vi "ESP32 Continuous Serial Write and Read.vi"() -> ()   [LabVIEW 2025]
doc: "This example performs writes and reads on a serial port, as directed by the user. You can press the Write and Read buttons, and change the Read Count, while the example is running.\n\nThe parameters set for the serial port must match the parameters of the connected instrument or device. In this example, the Read Count parameter specifies the number of bytes that the serial port reads. If there were more bytes at the port than the specified number, those bytes would not be read. If there were less bytes at the port than the specified number, you would receive a timeout error.\n\nThis example expands upon the flow control options for XON and XOFF, allowing the user to choose those control characters. Also, the user can enable or disable a termination character. Some devices require a termination character in order to identify the end of command strings. Some devices send a termination character to signify the end of data to be read. This example shows how you can end the Read operation once a termination character is detected in the buffer and/or append a termination character at the end of the Write data."
uses:
  Serial - Settings.ctl
  Control 1.ctl
  ESP32-PSOC-State Machine-1.ctl
  <vilib>/Instr/_visa.llb/VISA Flush IO Buffer Mask.ctl
  <vilib>/Instr/_visa.llb/VISA Configure Serial Port (Instr).vi
panel:
  in  "Command R":bool
  out "error":bool
  out "Connected":bool
  out "Serial Settings:Number of Bytes at Serial Port":u32
  out "Response 2":string
  in  "Command B":bool
  in  "Command A":bool
  in  "Toggle LED":bool
  in  "Enum":T1
  in  "Termination Character":u8=10 format="%.0x"
  in  "End Write on Termination Character?":bool=TRUE
  in  "Stop":bool
  out "Read Count":u32=1000
  out "Response":string
  in  "XON/XOFF Characters":T2={"XON"=enum."DC1", "XOFF"=enum."DC3"}
  in  "Serial Settings":T3={"baud rate"=115200, "data bits"=8, "parity"=enum."None", "stop bits"=10, "flow control"=0} {"flow control" items=["None"=0, "XON/XOFF"=1, "RTS/CTS"=2, "DTR/DSR"=4]; "stop bits" items=["1.0"=10, "1.5"=15, "2.0"=20]; "data bits" min=5 max=8 step=1; "baud rate" items=["75"=75, "110"=110, "134"=134, "150"=150, "300"=300, "600"=600, "1200"=1200, "1800"=1800, "2400"=2400, "4800"=4800, "7200"=7200, "9600"=9600, "14400"=14400, "19200"=19200, "28800"=28800, "38400"=38400, "56000"=56000, "57600"=57600, "115200"=115200, "128000"=128000, "230400"=230400]}
  in  "End Read on Termination Character?":bool=TRUE
  in  "VISA resource name":refnum<visa-resource-name>="COM3"
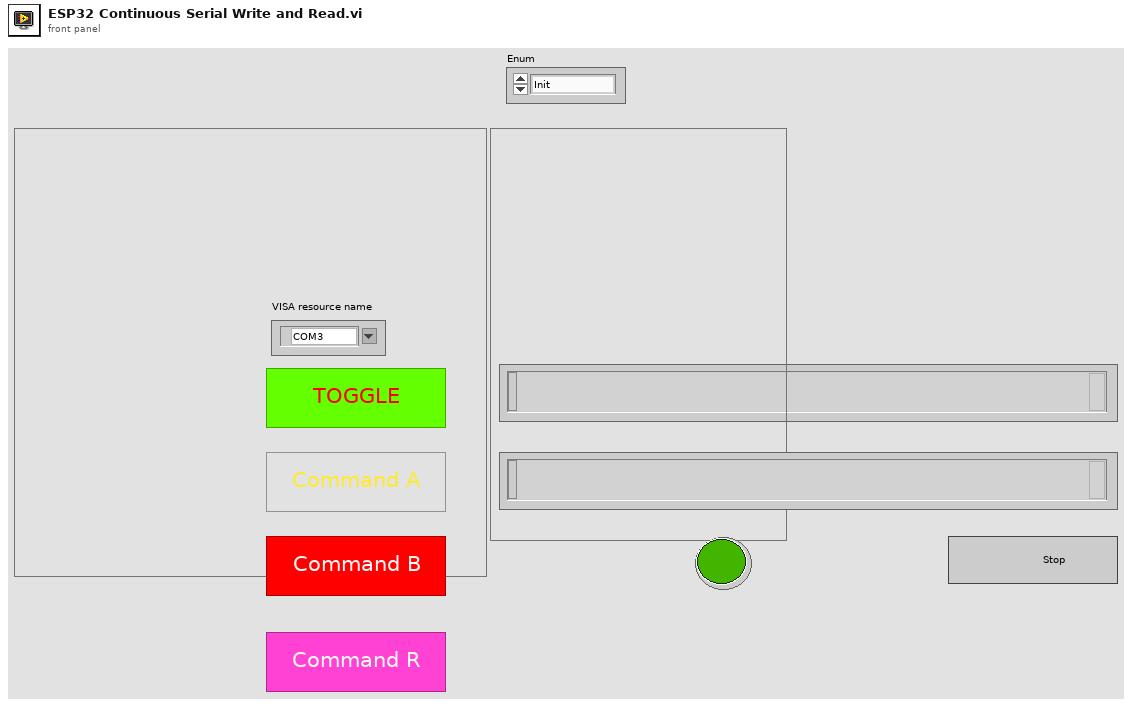
[diagram p1: front panel]
types:
  T1 = typedef "ESP32-PSOC-State Machine-1.ctl" = enum8{"Init", "Connect", "idle", "send", "wait", "receive", "que", "error", "exit"}
  T2 = typedef "Control 1.ctl" = cluster{"XON":enum16{"NUL", "SOH", "STX", "ETX", "EOT", "ENQ", "ACK", "BEL", "BS", "HT", "LF", "VT", "FF", "CR", "SO", "SI", "DLE", "DC1", "DC2", "DC3", "DC4", "NAK", "SYN", "ETB", "CAN", "EM", "SUB", "ESC", "FS", "GS", "RS", "US", "SP", "!", "\"", "#", "$", "%", "&", "'", "(", ")", "*", "+", ",", "- (-)", ".", "/", "0", "1", "2", "3", "4", "5", "6", "7", "8", "9", ":", ";", "<", "=", ">", "?", "@", "A", "B", "C", "D", "E", "F", "G", "H", "I", "J", "K", "L", "M", "N", "O", "P", "Q", "R", "S", "T", "U", "V", "W", "X", "Y", "Z", "[", "\\", "]", "^", "_", "`", "a", "b", "c", "d", "e", "f", "g", "h", "i", "j", "k", "l", "m", "n", "o", "p", "q", "r", "s", "t", "u", "v", "w", "x", "y", "z", "{", "|", "}", "~"}, "XOFF":enum16{"NUL", "SOH", "STX", "ETX", "EOT", "ENQ", "ACK", "BEL", "BS", "HT", "LF", "VT", "FF", "CR", "SO", "SI", "DLE", "DC1", "DC2", "DC3", "DC4", "NAK", "SYN", "ETB", "CAN", "EM", "SUB", "ESC", "FS", "GS", "RS", "US", "SP", "!", "\"", "#", "$", "%", "&", "'", "(", ")", "*", "+", ",", "- (-)", ".", "/", "0", "1", "2", "3", "4", "5", "6", "7", "8", "9", ":", ";", "<", "=", ">", "?", "@", "A", "B", "C", "D", "E", "F", "G", "H", "I", "J", "K", "L", "M", "N", "O", "P", "Q", "R", "S", "T", "U", "V", "W", "X", "Y", "Z", "[", "\\", "]", "^", "_", "`", "a", "b", "c", "d", "e", "f", "g", "h", "i", "j", "k", "l", "m", "n", "o", "p", "q", "r", "s", "t", "u", "v", "w", "x", "y", "z", "{", "|", "}", "~"}}
  T3 = typedef "Serial - Settings.ctl" = cluster{"baud rate":u32, "data bits":u16, "parity":enum16{"None", "Odd", "Even", "Mark", "Space"}, "stop bits":u16, "flow control":u16}
  T4 = enum16{"NUL", "SOH", "STX", "ETX", "EOT", "ENQ", "ACK", "BEL", "BS", "HT", "LF", "VT", "FF", "CR", "SO", "SI", "DLE", "DC1", "DC2", "DC3", "DC4", "NAK", "SYN", "ETB", "CAN", "EM", "SUB", "ESC", "FS", "GS", "RS", "US", "SP", "!", "\"", "#", "$", "%", "&", "'", "(", ")", "*", "+", ",", "- (-)", ".", "/", "0", "1", "2", "3", "4", "5", "6", "7", "8", "9", ":", ";", "<", "=", ">", "?", "@", "A", "B", "C", "D", "E", "F", "G", "H", "I", "J", "K", "L", "M", "N", "O", "P", "Q", "R", "S", "T", "U", "V", "W", "X", "Y", "Z", "[", "\\", "]", "^", "_", "`", "a", "b", "c", "d", "e", "f", "g", "h", "i", "j", "k", "l", "m", "n", "o", "p", "q", "r", "s", "t", "u", "v", "w", "x", "y", "z", "{", "|", "}", "~"}
  T5 = typedef "VISA Flush IO Buffer Mask.ctl" = u16
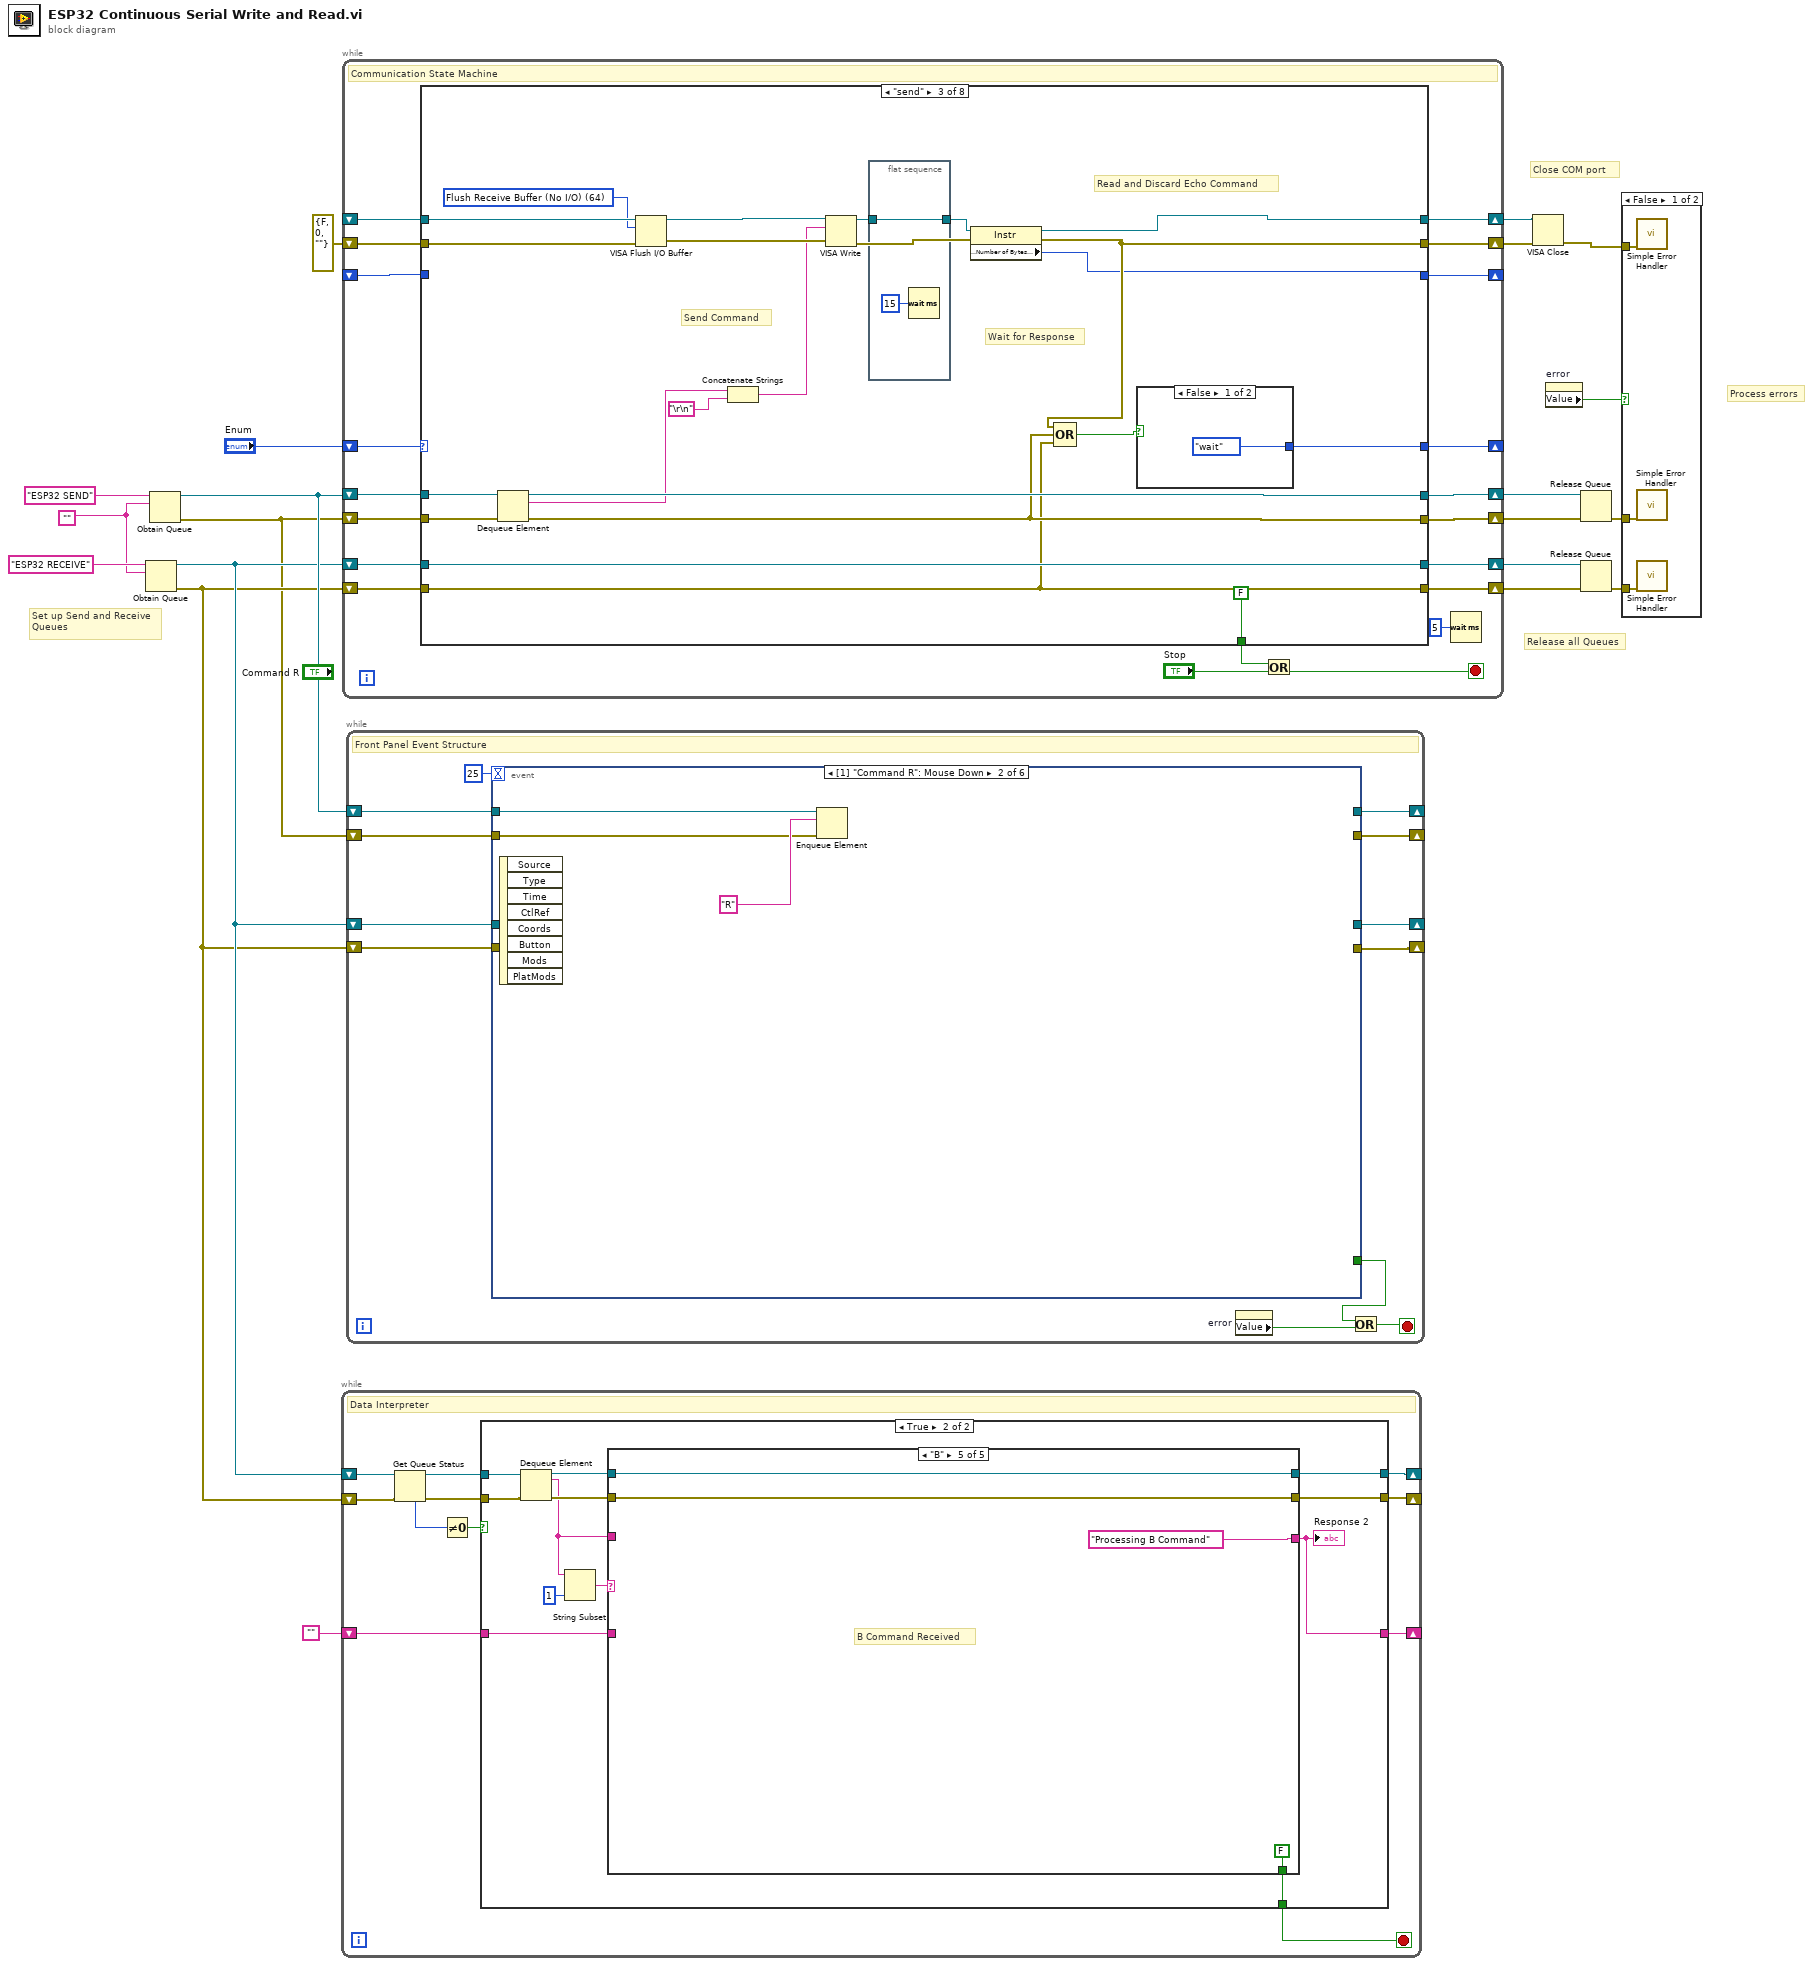
[diagram p0: block diagram]
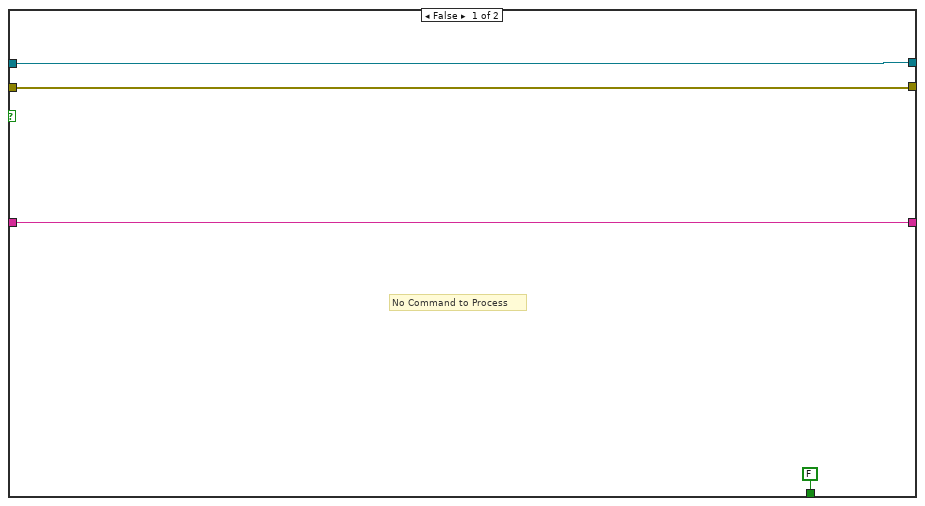
[diagram p3: hidden frame]
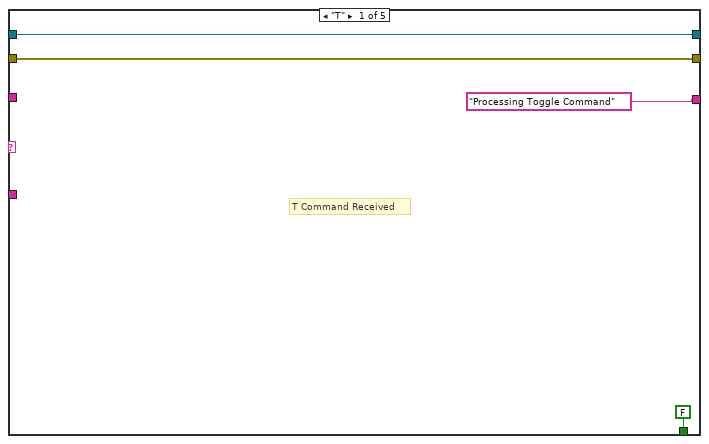
[diagram p4: hidden frame]
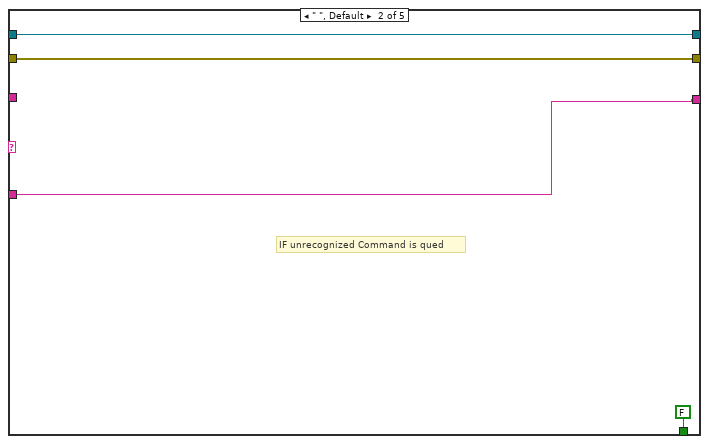
[diagram p5: hidden frame]
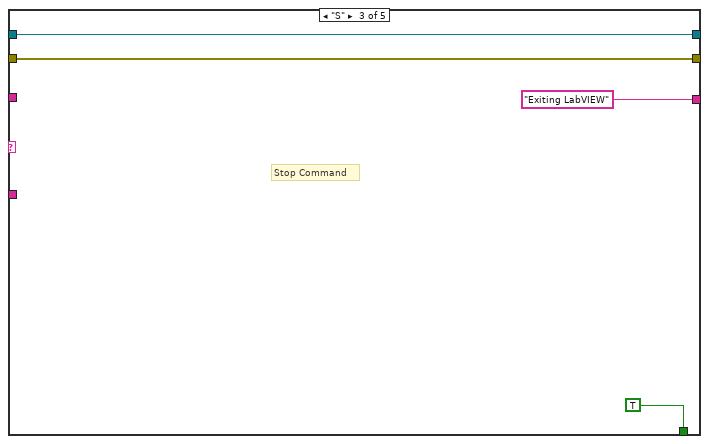
[diagram p6: hidden frame]
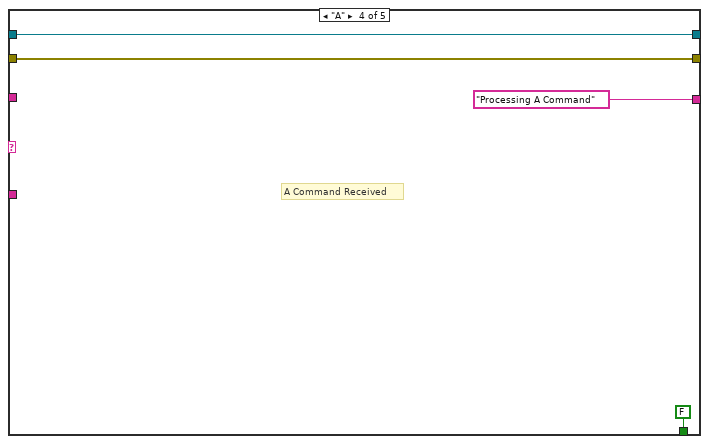
[diagram p7: hidden frame]
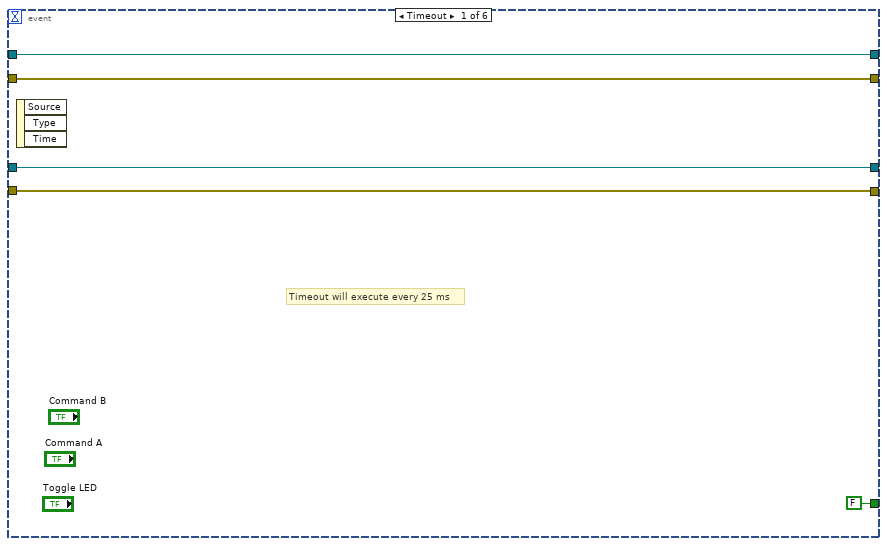
[diagram p8: hidden frame]
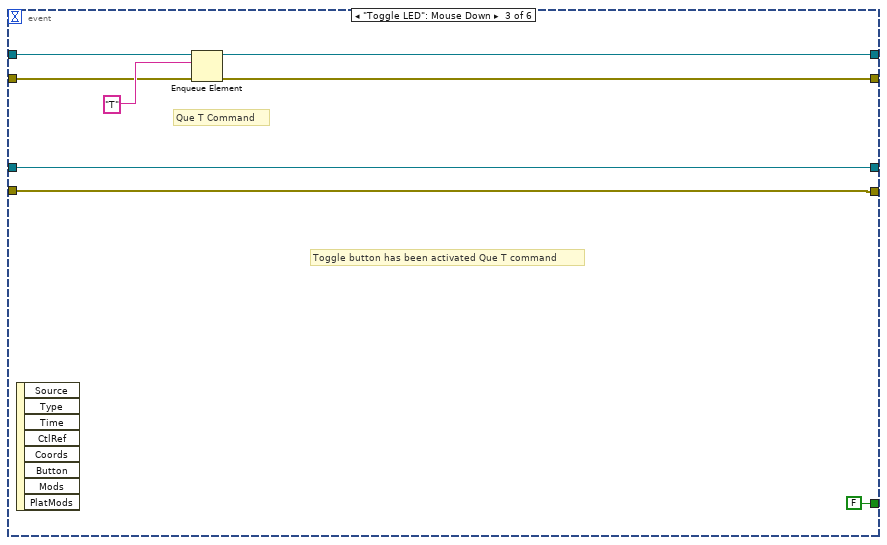
[diagram p9: hidden frame]
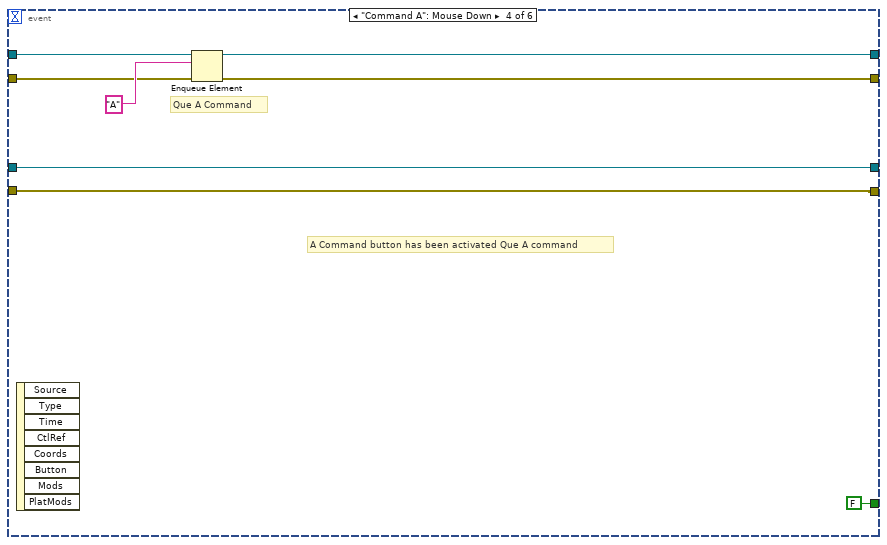
[diagram p10: hidden frame]
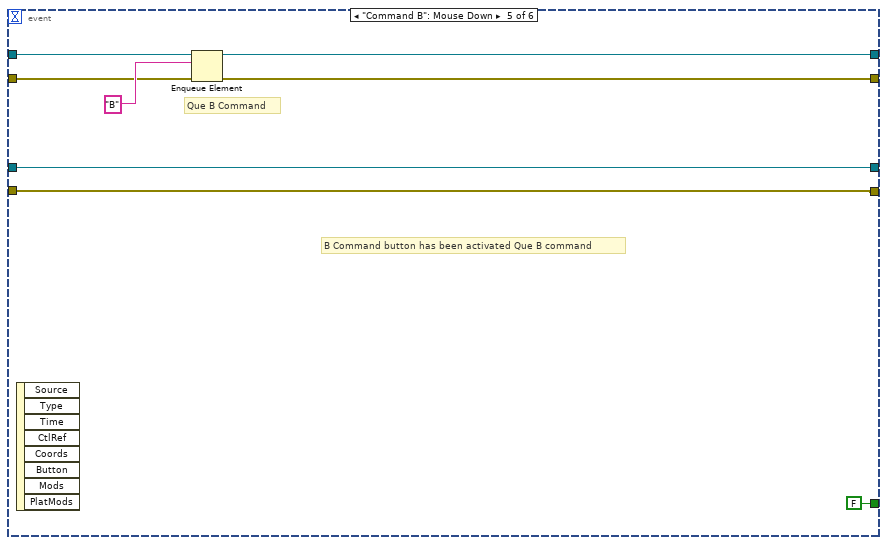
[diagram p11: hidden frame]
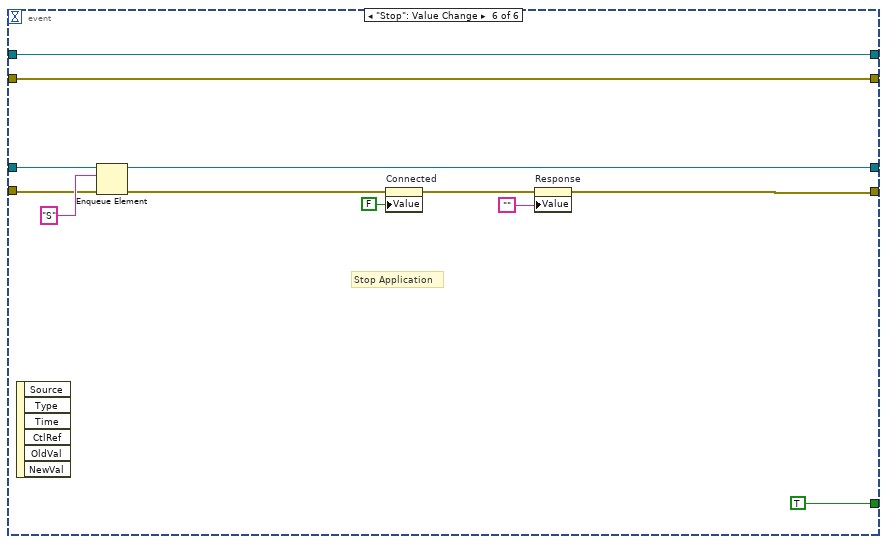
[diagram p12: hidden frame]
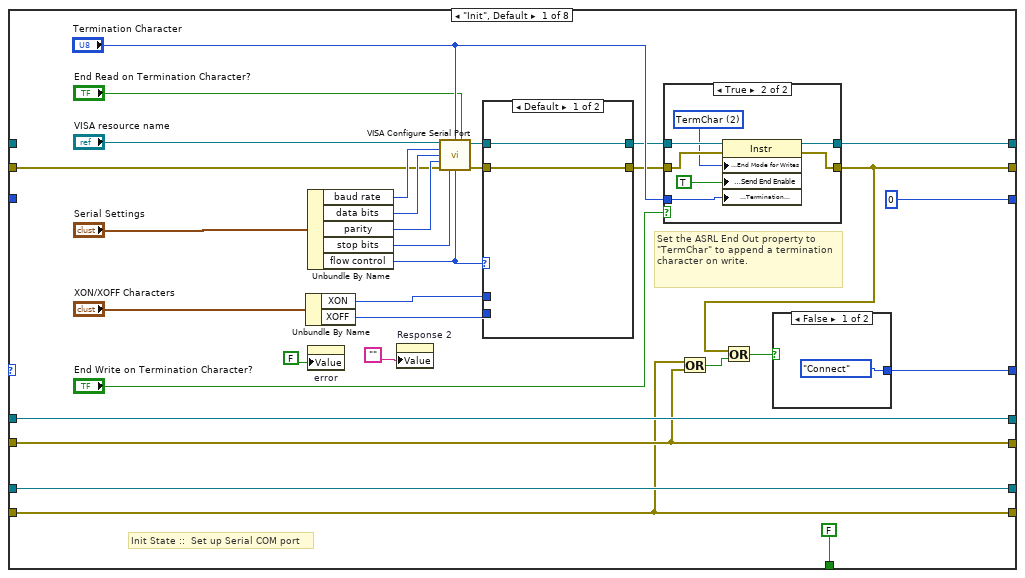
[diagram p13: hidden frame]
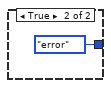
[diagram p14: hidden frame]
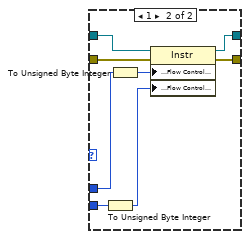
[diagram p16: hidden frame]
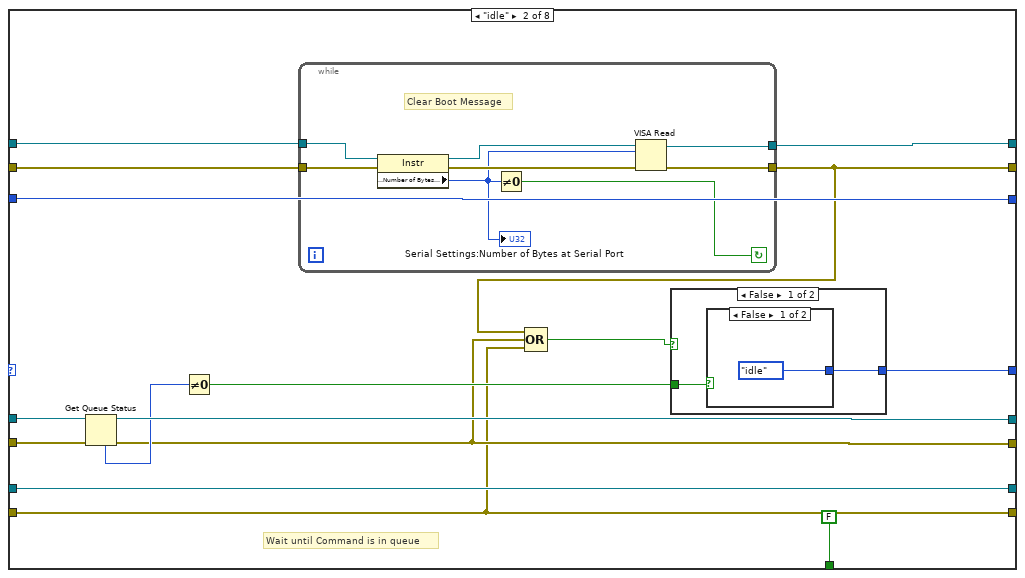
[diagram p17: hidden frame]
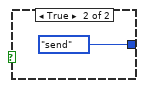
[diagram p18: hidden frame]
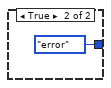
[diagram p19: hidden frame]
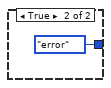
[diagram p20: hidden frame]
diagram:
  w10 = ""
  # "Process errors"
  # "Release all Queues"
  # "Close COM port"
  # "Set up Send and Receive\nQueues"
  n1 = Obtain Queue(name (unnamed)="ESP32 RECEIVE", element data type=w10) -> (queue out=w9:refnum<queue>, error out=w8:errorcluster)  [unwired: 3 in, 1 out]
  n2 = Obtain Queue(name (unnamed)="ESP32 SEND", element data type=w10) -> (queue out=w12:refnum<queue>, error out=w2:errorcluster)  [unwired: 3 in, 1 out]
  n3 = while {
    shift-right: [w25] -> _
    shift-left: w9 -> [w31]
    shift-right: [w24] -> _
    shift-left: w8 -> [w30]
    shift-right: [w22] -> _
    shift-left: "" -> [w21]
    stop <- w23 stop-if-true
    # "Data Interpreter"
    n4 = Get Queue Status(queue=w31, error in (no error)=w30) -> (queue out=w27:refnum<queue>, error out=w26:errorcluster, # elements in queue=w29:i32)  [unwired: 1 in, 5 out]
    n5 = Not Equal To 0?(x=w29) -> (x != 0?=w28:bool)
    n6 = case shown="True" w28 {
      tunnel: w27 -> [w35 w47]
      tunnel: w26 -> [w34 w46]
      tunnel: [w35 w41] -> w25
      tunnel: [w34 w40] -> w24
      tunnel: [FALSE w39] -> w23
      tunnel: [w32 w37] -> w22
      tunnel: w21 -> [w32 w36]
      frame False {
        # "No Command to Process"
      }
      frame True {
        n7 = Dequeue Element(queue=w47, error in (no error)=w46) -> (queue out=w45:refnum<queue>, element=w38:string, error out=w44:errorcluster)  [unwired: 1 in, 1 out]
        n8 = String Subset(string=w38, length (rest)=1 ("length (rest)")) -> (substring=w42:string)  [unwired: 1 in]
        n9 = case shown="\"B\"" w42 {
          tunnel: w45 -> [w51 w55 w59 w63 w67]
          tunnel: w44 -> [w50 w54 w58 w62 w66]
          tunnel: [w51 w55 w59 w63 w67] -> w41
          tunnel: [w50 w54 w58 w62 w66] -> w40
          tunnel: w38 -> [_ _ _ _ _]
          tunnel: [FALSE FALSE TRUE FALSE FALSE] -> w39
          tunnel: ["Processing Toggle Command" w52 "Exiting LabVIEW" "Processing A Command" "Processing B Command"] -> w37
          tunnel: w36 -> [_ w52 _ _ _]
          frame "T" {
            # "T Command Received"
          }
          frame " ", Default {
            # "IF unrecognized Command is qued"
          }
          frame "S" {
            # "Stop Command"
          }
          frame "A" {
            # "A Command Received"
          }
          frame "B" {
            # "B Command Received"
          }
        }
        "Response 2" <- w37
      }
    }
  }
  n10 = while {
    shift-right: [w79] -> w20
    shift-left: w12 -> [w87]
    shift-right: [w78] -> w18
    shift-left: w2 -> [w86]
    shift-right: [w77] -> w19
    shift-left: w9 -> [w85]
    shift-right: [w76] -> w15
    shift-left: w8 -> [w84]
    shift-right: [w71] -> _
    shift-left: "Enum" -> [w70]
    shift-right: [w83] -> w14
    shift-left: _ -> [w80]
    shift-right: [w82] -> w13
    shift-left: errorcluster {"status"=FALSE, "code"=0, "source"=""} ("error out") -> [w81]
    shift-right: [w75] -> _
    shift-left: _ -> [w74]
    stop <- w69 stop-if-true
    # "Communication State Machine"
    n11 = case shown="\"send\"" w70 {
      selector: w70 -> [_ _ _ _ _ _ w282 _]
      tunnel: [w117 w153 w189 w206 w244 w266 w281 w304] -> w79
      tunnel: [w91 w143 w181 w200 w227 w263 w280 w303] -> w78
      tunnel: [w97 w151 w182 w209 w245 ESP32-PSOC-State_Machine-1."exit" ("Enum") w282 ESP32-PSOC-State_Machine-1."idle" ("Enum")] -> w71
      tunnel: w87 -> [w117 w155 w191 w206 w244 w266 w281 w304]
      tunnel: w86 -> [w91 w154 w190 w200 w227 w263 w280 w303]
      tunnel: w85 -> [w118 w149 w188 w203 w239 w265 w279 w302]
      tunnel: w84 -> [w90 w142 w180 w199 w226 w262 w270 w301]
      tunnel: [w99 w146 w177 w208 w235 w268 w285 w306] -> w83
      tunnel: [w93 w144 w175 w201 w228 w264 w284 w307] -> w82
      tunnel: w81 -> [w95 w145 w185 w207 w230 w264 w284 w308]
      tunnel: w80 -> [_ w147 w187 w197 w242 w268 w285 w309]
      tunnel: [w118 w149 w188 w203 w237 w265 w277 w302] -> w77
      tunnel: [w90 w142 w180 w199 w238 w262 w273 w301] -> w76
      tunnel: [u32 0 ("Bytes at Port") w148 w169 w205 w240 w267 w283 w305] -> w75
      tunnel: w74 -> [_ w148 _ _ w218 w267 w283 w305]
      tunnel: [FALSE FALSE FALSE FALSE FALSE FALSE TRUE FALSE] -> w68
      frame "Init", Default {
        # "Init State ::  Set up Serial COM port"
        # "Set the ASRL End Out property to \"TermChar\" to append a termination character on write."
        n12 = Unbundle By Name("XON/XOFF Characters") -> ("XON"=w111:T4, "XOFF"=w112:T4)
        n13 = Unbundle By Name("Serial Settings") -> ("baud rate"=w107:u32, "data bits"=w106:u16, "parity"=w105:enum16{"None", "Odd", "Even", "Mark", "Space"}, "stop bits"=w104:u16, "flow control"=w110:u16)
        n14 = property on="error" class="Bool (strict)"("Value"=FALSE ("error")) -> ()  [unwired: 2 in, 2 out]
        n15 = property on="Response 2" class="Str"("Value"="") -> ()  [unwired: 2 in, 2 out]
        n16 = call-poly "VISA Configure Serial Port"("VISA resource name"="VISA resource name", "termination char\n(0xA = '\\n' = LF)"="Termination Character", "Enable Termination\nChar (T)"="End Read on Termination Character?", "baud rate (9600)"=w107, "data bits (8)"=w106, "parity (0:none)"=w105, "error in (no error)"=w95, "stop bits (10: 1 bit)"=w104, "flow control (0:none)"=w110) -> ("VISA resource name out"=w103:refnum<visa-resource-name>, "error out"=w102:errorcluster)  [unwired: 1 in, 4 out]
        n17 = case shown="Default" w110 {
          tunnel: [w130 w139] -> w113
          tunnel: [w131 w138] -> w114
          tunnel: w102 -> [w130 w137]
          tunnel: w103 -> [w131 w136]
          tunnel: w111 -> [_ w135]
          tunnel: w112 -> [_ w134]
          frame Default {
          }
          frame 1 {
            n18 = To Unsigned Byte Integer(number=w134) -> (unsigned 8bit integer=w133:u8)
            n19 = To Unsigned Byte Integer(number=w135) -> (unsigned 8bit integer=w132:u8)
            n20 = property class="Instr"(reference=w136, error in=w137, "Serial Settings:Flow Control XON Character"=w132, "Serial Settings:Flow Control XOFF Character"=w133) -> (reference out=w138:refnum<visa-resource-name>, error out=w139:errorcluster)
          }
        }
        n21 = case shown="True" "End Write on Termination Character?" {
          tunnel: w114 -> [w121 w129]
          tunnel: w113 -> [w122 w128]
          tunnel: [w121 w127] -> w99
          tunnel: [w122 w126] -> w93
          tunnel: "Termination Character" -> [_ w124]
          frame False {
          }
          frame True {
            w125 = u16 2 items=["None", "LastBit", "TermChar", "Break"] ("Serial Settings:Serial End Mode for Writes")
            n22 = property class="Instr"(reference=w129, error in=w128, "Serial Settings:End Mode for Writes"=w125, "Message Based Settings:Send End Enable"=TRUE, "Message Based Settings:Termination Character"=w124) -> (reference out=w127:refnum<visa-resource-name>, error out=w126:errorcluster)
          }
        }
        n23 = Or(x=w90, y=w91) -> (x .or. y?=w92:bool)
        n24 = Or(x=w93, y=w92) -> (x .or. y?=w94:bool)
        n25 = case shown="False" w94 {
          tunnel: [ESP32-PSOC-State_Machine-1."Connect" ("Enum") ESP32-PSOC-State_Machine-1."error" ("Enum")] -> w97
          frame False {
          }
          frame True {
          }
        }
      }
      frame "idle" {
        # "Wait until Command is in queue"
        n26 = Get Queue Status(queue=w155, error in (no error)=w154) -> (queue out=w153:refnum<queue>, error out=w143:errorcluster, # elements in queue=w152:i32)  [unwired: 1 in, 5 out]
        n27 = Not Equal To 0?(x=w152) -> (x != 0?=w150:bool)
        n28 = while {
          tunnel: w147 -> [w168]
          tunnel: [w164] -> w146
          tunnel: w145 -> [w167]
          tunnel: [w162] -> w144
          stop <- w166 continue-if-true
          # "Clear Boot Message"
          n29 = property class="Instr"(reference=w168, error in=w167) -> (reference out=w165:refnum<visa-resource-name>, error out=w163:errorcluster, "Serial Settings:Number of Bytes at Serial Port"=w161:u32)
          "Serial Settings:Number of Bytes at Serial Port" <- w161
          n30 = Not Equal To 0?(x=w161) -> (x != 0?=w166:bool)
          n31 = VISA Read(VISA resource name=w165, byte count=w161, error in (no error)=w163) -> (VISA resource name out=w164:refnum<visa-resource-name>, error out=w162:errorcluster)  [unwired: 2 out]
        }
        n32 = Compound Arithmetic op=OR(w144, w143, w142) -> (w141:bool)
        n33 = case shown="False" w141 {
          tunnel: [w157 ESP32-PSOC-State_Machine-1."error" ("Enum")] -> w151
          tunnel: w150 -> [w156 _]
          frame False {
            n34 = case shown="False" w156 {
              tunnel: [ESP32-PSOC-State_Machine-1."idle" ("Enum") ESP32-PSOC-State_Machine-1."send" ("Enum")] -> w157
              frame False {
              }
              frame True {
              }
            }
          }
          frame True {
          }
        }
      }
      frame "send" {
        w183 = T5 64 items=["Flush Receive Buffer"=16, "Write Transmit Buffer to Device"=32, "Flush Receive Buffer (No I/O)"=64, "Flush Transmit Buffer"=128] ("Mask")
        # "Read and Discard Echo Command"
        # "Wait for Response"
        # "Send Command"
        n35 = Dequeue Element(queue=w191, error in (no error)=w190) -> (queue out=w189:refnum<queue>, element=w173:string, error out=w181:errorcluster)  [unwired: 1 in, 1 out]
        n36 = VISA Flush I/O Buffer(VISA resource name=w187, mask (16)=w183, error in (no error)=w185) -> (VISA resource name out=w186:refnum<visa-resource-name>, error out=w184:errorcluster)
        n37 = Concatenate Strings(w173, "\r\n") -> (w172:string)
        n38 = VISA Write(VISA resource name=w186, write buffer=w172, error in (no error)=w184) -> (VISA resource name out=w171:refnum<visa-resource-name>, error out=w176:errorcluster)  [unwired: 1 out]
        n39 = flat-sequence {
          tunnel: w171 -> [w193]
          tunnel: [w193] -> w170
          frame #0 {
            n40 = Wait (ms)(milliseconds to wait=u32 15) -> ()  [unwired: 1 out]
          }
        }
        n41 = property class="Instr"(reference=w170, error in=w176) -> (reference out=w177:refnum<visa-resource-name>, error out=w175:errorcluster, "Serial Settings:Number of Bytes at Serial Port"=w169:u32)
        n42 = Compound Arithmetic op=OR(w175, w181, w180) -> (w179:bool)
        n43 = case shown="False" w179 {
          tunnel: [ESP32-PSOC-State_Machine-1."wait" ("Enum") ESP32-PSOC-State_Machine-1."error" ("Enum")] -> w182
          frame False {
          }
          frame True {
          }
        }
      }
      frame "wait" {
        # "Wait for actual Response"
        n44 = flat-sequence {
          tunnel: w197 -> [w211]
          tunnel: [w211] -> w196
          frame #0 {
            n45 = Wait (ms)(milliseconds to wait=u32 15) -> ()  [unwired: 1 out]
          }
        }
        n46 = property class="Instr"(reference=w196, error in=w207) -> (reference out=w208:refnum<visa-resource-name>, error out=w201:errorcluster, "Serial Settings:Number of Bytes at Serial Port"=w205:u32)
        n47 = Not Equal To 0?(x=w205) -> (x != 0?=w204:bool)
        n48 = Compound Arithmetic op=OR(w201, w200, w199) -> (w202:bool)
        n49 = case shown="False" w202 {
          tunnel: [w213 ESP32-PSOC-State_Machine-1."error" ("Enum")] -> w209
          tunnel: w204 -> [w212 _]
          frame False {
            n50 = case shown="True" w212 {
              tunnel: [ESP32-PSOC-State_Machine-1."wait" ("Enum") ESP32-PSOC-State_Machine-1."receive" ("Enum")] -> w213
              frame False {
              }
              frame True {
              }
            }
          }
          frame True {
          }
        }
      }
      frame "receive" {
        # "Process Response and Display"
        # "Read Response"
        n51 = VISA Read(VISA resource name=w242, byte count=w218, error in (no error)=w230) -> (VISA resource name out=w236:refnum<visa-resource-name>, read buffer=w232:string, return count=w217:u32, error out=w241:errorcluster)
        n52 = String To Byte Array(string=w232) -> (unsigned byte array=w231:u8[])
        n53 = property class="Instr"(reference=w236, error in=w241) -> (reference out=w235:refnum<visa-resource-name>, error out=w229:errorcluster, "Serial Settings:Number of Bytes at Serial Port"=w240:u32)
        n54 = Index Array(array=w231, index=0) -> (element=w223:u8)
        n55 = Equal?(x=w223, y=u8 13) -> (x = y?=w221:bool)
        n56 = Equal?(x=w223, y=u8 10) -> (x = y?=w220:bool)
        n57 = Not Or(1:w220, 2:w221) -> (0:w219:bool)
        n58 = Not Equal To 0?(x=w240) -> (x != 0?=w243:bool)
        n59 = case shown="True" w219 {
          tunnel: w231 -> [_ w252]
          tunnel: w229 -> [w251 w254]
          tunnel: [w251 w253] -> w228
          tunnel: w217 -> [_ _]
          frame False {
          }
          frame True {
            (unwired) 1 ("length")
            (unwired) 0 ("index")
            n60 = property on="Response" class="Str"(error in=w254, "Value"="") -> (error out=w256:errorcluster)  [unwired: 1 in, 1 out]
            n61 = Byte Array To String(unsigned byte array=w252) -> (string=w255:string)
            n62 = property on="Response" class="Str"(error in=w256, "Value"=w255) -> (error out=w253:errorcluster)  [unwired: 1 in, 1 out]
          }
        }
        n63 = Compound Arithmetic op=OR(w228, w227, w226) -> (w225:bool)
        n64 = Enqueue Element(queue=w239, element=w232, error in (no error)=w226) -> (queue out=w237:refnum<queue>, error out=w238:errorcluster)  [unwired: 1 in, 1 out]
        n65 = case shown="False" w225 {
          tunnel: [w247 ESP32-PSOC-State_Machine-1."error" ("Enum")] -> w245
          tunnel: w243 -> [w246 _]
          frame False {
            n66 = case shown="False" w246 {
              tunnel: [ESP32-PSOC-State_Machine-1."idle" ("Enum") ESP32-PSOC-State_Machine-1."receive" ("Enum")] -> w247
              frame False {
              }
              frame True {
              }
            }
          }
          frame True {
          }
        }
        "Read Count" <- w218
      }
      frame "error" {
        # "Process any error"
        n67 = Build Array(w264, w263, w262) -> (w261:errorcluster[])
        n68 = for {
          tunnel: w261 -> [w269] mode=indexing
          n69 = call <vilib>:"General Error Handler.vi"("error in (no error)"=w269) -> ()  [unwired: 10 in, 5 out]
        }
        "error" <- TRUE ("error")
      }
      frame "exit" {
        # "Exit due to error"
        n70 = Enqueue Element(queue=w279, element="S", error in (no error)=w270) -> (queue out=w277:refnum<queue>, error out=w275:errorcluster)  [unwired: 1 in, 1 out]
        n71 = property on="Connected" class="Bool (strict)"(error in=w275, "Value"=FALSE ("Connected")) -> (error out=w274:errorcluster)  [unwired: 1 in, 1 out]
        n72 = property on="Response" class="Str"(error in=w274, "Value"="") -> (error out=w273:errorcluster)  [unwired: 1 in, 1 out]
      }
      frame "Connect" {
        # "Validating connection"
        # "Send ID to validate connection"
        # "Clear any residual characters"
        n73 = while {
          shift-right: [w333] -> w297
          shift-left: w308 -> [w339]
          shift-right: [w332] -> w298
          shift-left: w309 -> [w338]
          stop <- w337 continue-if-true
          n74 = property class="Instr"(reference=w338, error in=w339) -> (reference out=w335:refnum<visa-resource-name>, error out=w334:errorcluster, "Bytes at Port"=w331:u32)
          n75 = VISA Read(VISA resource name=w335, byte count=w331, error in (no error)=w334) -> (VISA resource name out=w332:refnum<visa-resource-name>, read buffer=w330:string, error out=w333:errorcluster)  [unwired: 1 out]
          n76 = Wait (ms)(milliseconds to wait=u32 5) -> ()  [unwired: 1 out]
          n77 = Search/Split String(string=w330, search string/char (-)="Commands") -> (match + rest of string=w328:string)  [unwired: 1 in, 2 out]
          n78 = String Length(string=w328) -> (length=w327:i32)
          n79 = Equal To 0?(x=w327) -> (x = 0?=w337:bool)
        }
        n80 = Concatenate Strings("I" ("write buffer"), "\r\n") -> (w286:string)
        n81 = VISA Write(VISA resource name=w298, write buffer=w286, error in (no error)=w297) -> (VISA resource name out=w292:refnum<visa-resource-name>, error out=w296:errorcluster)  [unwired: 1 out]
        n82 = flat-sequence {
          tunnel: w292 -> [w326]
          tunnel: [w326] -> w291
          frame #0 {
            n83 = Wait (ms)(milliseconds to wait=u32 5) -> ()  [unwired: 1 out]
          }
        }
        n84 = property class="Instr"(reference=w291, error in=w296) -> (reference out=w294:refnum<visa-resource-name>, error out=w295:errorcluster, "Bytes at Port"=w293:u32)
        n85 = VISA Read(VISA resource name=w294, byte count=w293, error in (no error)=w295) -> (VISA resource name out=w289:refnum<visa-resource-name>, error out=w290:errorcluster)  [unwired: 2 out]
        n86 = while {
          shift-right: [w313] -> w307
          shift-left: w290 -> [w319]
          shift-right: [w314] -> w306
          shift-left: w289 -> [w312]
          stop <- w310 stop-if-true
          n87 = flat-sequence {
            tunnel: w312 -> [w324]
            tunnel: [w324] -> w311
            frame #0 {
              n88 = Wait (ms)(milliseconds to wait=u32 15) -> ()  [unwired: 1 out]
            }
          }
          n89 = property class="Instr"(reference=w311, error in=w319) -> (reference out=w317:refnum<visa-resource-name>, error out=w318:errorcluster, "Bytes at Port"=w316:u32)
          n90 = VISA Read(VISA resource name=w317, byte count=w316, error in (no error)=w318) -> (VISA resource name out=w314:refnum<visa-resource-name>, read buffer=w315:string, error out=w313:errorcluster)  [unwired: 1 out]
          n91 = Search/Split String(string=w315, search string/char (-)="ESP32") -> (match + rest of string=w321:string)  [unwired: 1 in, 2 out]
          n92 = String Length(string=w321) -> (length=w320:i32)
          n93 = Not Equal To 0?(x=w320) -> (x != 0?=w310:bool)
          "Connected" <- w310
        }
      }
    }
    n94 = Or(x=w68, y="Stop") -> (x .or. y?=w69:bool)
    n95 = Wait (ms)(milliseconds to wait=u32 5) -> ()  [unwired: 1 out]
  }
  n96 = while {
    shift-right: [w348] -> _
    shift-left: w12 -> [w349]
    shift-right: [w347] -> _
    shift-left: w2 -> [w350]
    shift-right: [w343] -> _
    shift-left: w9 -> [w346]
    shift-right: [w344] -> _
    shift-left: w8 -> [w345]
    stop <- w340 stop-if-true
    # "Front Panel Event Structure"
    n97 = event shown="[1] \"Command R\": Mouse Down" {
      selector: _ -> [_ _ _ _ _ _]
      dyn-events: _ -> [_ _ _ _ _ _]
      timeout: 25 -> [_ _ _ _ _ _]
      tunnel: w350 -> [w354 w357 w365 w373 w381 w393]
      tunnel: w349 -> [w355 w358 w367 w375 w383 w394]
      tunnel: [w355 _ w364 w372 w380 w394] -> w348
      tunnel: [w354 _ w363 w371 w379 w393] -> w347
      tunnel: [FALSE _ FALSE FALSE FALSE TRUE] -> w342
      tunnel: w346 -> [w353 _ w361 w369 w377 w392]
      tunnel: w345 -> [w352 _ w360 w368 w376 w390]
      tunnel: [w352 _ w360 w368 w376 w385] -> w344
      tunnel: [w353 _ w361 w369 w377 w389] -> w343
      event Timeout {
        # "Timeout will execute every 25 ms"
        n98 = event-data() -> ()  [unwired: 1 in, 3 out]
      }
      event "Command R": Mouse Down {
        n99 = event-data() -> ()  [unwired: 1 in, 8 out]
        n100 = Enqueue Element(queue=w358, element="R", error in (no error)=w357) -> ()  [unwired: 1 in, 3 out]
      }
      event "Toggle LED": Mouse Down {
        # "Que T Command"
        # "Toggle button has been activated Que T command"
        n101 = event-data() -> ()  [unwired: 1 in, 8 out]
        n102 = Enqueue Element(queue=w367, element="T", error in (no error)=w365) -> (queue out=w364:refnum<queue>, error out=w363:errorcluster)  [unwired: 1 in, 1 out]
      }
      event "Command A": Mouse Down {
        # "Que A Command"
        # "A Command button has been activated Que A command"
        n103 = event-data() -> ()  [unwired: 1 in, 8 out]
        n104 = Enqueue Element(queue=w375, element="A", error in (no error)=w373) -> (queue out=w372:refnum<queue>, error out=w371:errorcluster)  [unwired: 1 in, 1 out]
      }
      event "Command B": Mouse Down {
        # "Que B Command"
        # "B Command button has been activated Que B command"
        n105 = event-data() -> ()  [unwired: 1 in, 8 out]
        n106 = Enqueue Element(queue=w383, element="B", error in (no error)=w381) -> (queue out=w380:refnum<queue>, error out=w379:errorcluster)  [unwired: 1 in, 1 out]
      }
      event "Stop": Value Change {
        # "Stop Application"
        n107 = event-data() -> ()  [unwired: 1 in, 6 out]
        n108 = Enqueue Element(queue=w392, element="S", error in (no error)=w390) -> (queue out=w389:refnum<queue>, error out=w388:errorcluster)  [unwired: 1 in, 1 out]
        n109 = property on="Connected" class="Bool (strict)"(error in=w388, "Value"=FALSE ("Connected")) -> (error out=w386:errorcluster)  [unwired: 1 in, 1 out]
        n110 = property on="Response" class="Str"(error in=w386, "Value"="") -> (error out=w385:errorcluster)  [unwired: 1 in, 1 out]
      }
    }
    n111 = property on="error" class="Bool (strict)"() -> ("Value"=w341:bool)  [unwired: 2 in, 2 out]
    n112 = Or(x=w342, y=w341) -> (x .or. y?=w340:bool)
  }
  n113 = VISA Close(VISA resource name=w14, error in (no error)=w13) -> (error out=w5:errorcluster)
  n114 = property on="error" class="Bool (strict)"() -> ("Value"=w1:bool)  [unwired: 2 in, 2 out]
  n115 = Release Queue(queue=w20, error in (no error)=w18) -> (error out=w4:errorcluster)  [unwired: 1 in, 2 out]
  n116 = Release Queue(queue=w19, error in (no error)=w15) -> (error out=w3:errorcluster)  [unwired: 1 in, 2 out]
  n117 = case shown="False" w1 {
    tunnel: w5 -> [w398 _]
    tunnel: w4 -> [w397 _]
    tunnel: w3 -> [w396 _]
    frame False {
      n118 = call <vilib>:"Simple Error Handler.vi"("error in (no error)"=w398) -> ()  [unwired: 1 in, 8 out]
      n119 = call <vilib>:"Simple Error Handler.vi"("error in (no error)"=w397) -> ()  [unwired: 1 in, 8 out]
      n120 = call <vilib>:"Simple Error Handler.vi"("error in (no error)"=w396) -> ()  [unwired: 1 in, 8 out]
    }
    frame True {
    }
  }
